vi "FormatFloat.vi"(8 "error in (no error)":errorcluster, 10 "replace string (\".\")":string=".", 11 "float":dbl) -> (0 "error out":errorcluster, 3 "string":string)   [LabVIEW 2018, in "AnalysisPlugins.lvlib" / "PmuAnalysis.lvclass"]
uses:
  PmuAnalysis.lvclass
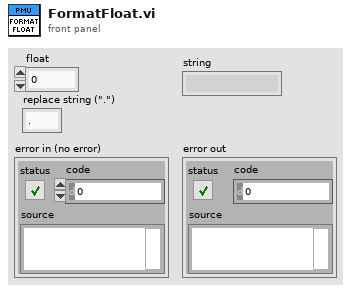
[diagram p1: front panel]
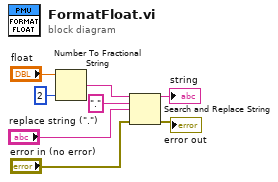
[diagram p0: block diagram]
diagram:
  n1 = Number To Fractional String(number="float", precision (6)=i16 2) -> (F-format string=w6:string)  [unwired: 2 in]
  n2 = Search and Replace String(input string=w6, search string=".", replace string="replace string (\".\")", error in="error in (no error)") -> (result string=→"string":string, error out=→"error out":errorcluster)  [unwired: 4 in, 2 out]
